vi "gfitsio-compute-lpixel.vi"(10 "dimension sizes of subset":i32[](array[numeric]), 11 "fpixel in":i32[](array[numeric])) -> (3 "lpixel":i32[](array[numeric]))   [LabVIEW 2021, in "gfitsio.lvlib"]
doc: "This VI comuputes the lpixel corresponding to the given fpixel and dimensions sizes."
uses:
  gfitsio.lvlib
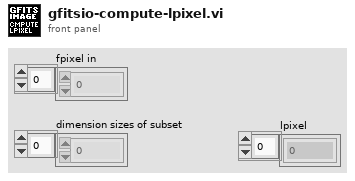
[diagram p1: front panel]
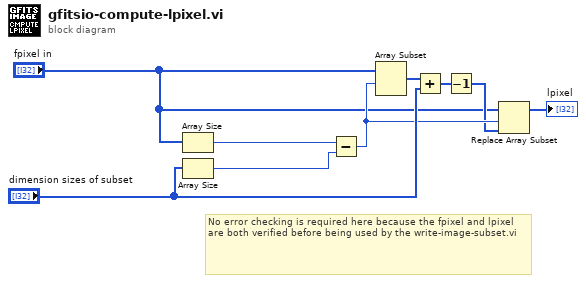
[diagram p0: block diagram]
diagram:
  # "No error checking is required here because the fpixel and lpixel are both verified before being used by the write-image-subset.vi"
  n1 = Array Size(array="fpixel in") -> (size(s)=w6:i32)
  n2 = Array Size(array="dimension sizes of subset") -> (size(s)=w7:i32)
  n3 = Subtract(x=w6, y=w7) -> (x-y=w8:i32)
  n4 = Array Subset(array="fpixel in", index=w8) -> (w2:i32[])  [unwired: 1 in]
  n5 = Add(x=w2, y="dimension sizes of subset") -> (x+y=w3:i32[])
  n6 = Decrement(x=w3) -> (x-1=w4:i32[])
  n7 = Replace Array Subset(array="fpixel in", new element=w4, index=w8) -> (→"lpixel":i32[])
